vi "Trigger Pulse Width.vi"(5 "Lower Limit":dbl, 6 "Upper Limit":dbl, 7 "Type":i32(ring) caption="Mode" items=["Inside Limits", "Outside Limits", "Less Than", "Greater Than", "Equal To", "Not Equal To"], 8 "error in":errorcluster, 9 "Level":dbl, 10 "Source":i32(ring) items=["TTL0", "TTL1", "TTL2", "TTL3", "TTL4", "TTL5", "TTL6", "TTL7", "ECL0", "ECL1", "Input Channel 1", "Input Channel 2", "Input Channel 3", "Input Channel 4", "Eternal Trigger Source", "STAR", "Manual Trigger", "Pattern"], 11 "Instrument Handle In":i32) -> (0 "error out":errorcluster, 3 "Instrument Handle Out":i32)   [LabVIEW 8.6, in "ZTScopeM.lvlib"]
doc: "Set the trigger type to pulse width and configure the pulse width trigger settings."
uses:
  ZTScopeM.lvlib
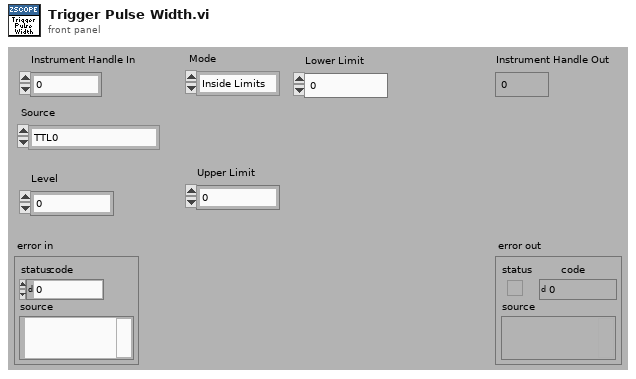
[diagram p1: front panel]
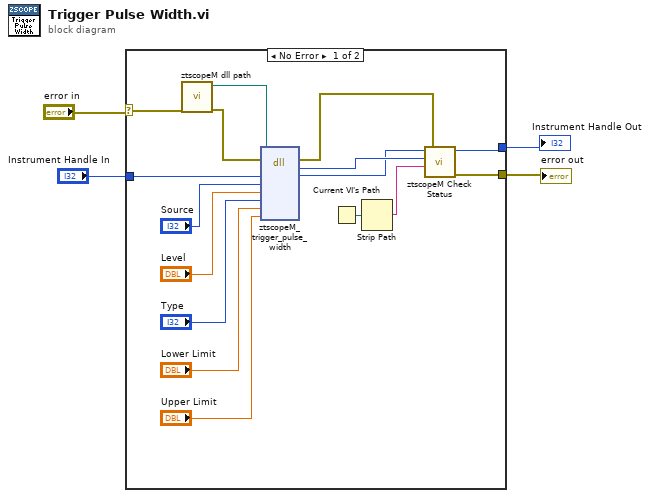
[diagram p0: block diagram]
diagram:
  n1 = case shown="No Error" "error in" {
    selector: "error in" -> [w8 w22]
    tunnel: [w9 w22] -> w2
    tunnel: "Instrument Handle In" -> [w20 w21]
    tunnel: [w10 w21] -> w1
    frame #0 {
      n2 = call "ztscopeM dll path.vi"("error in (no error)"=w8) -> ("error out"=w6:errorcluster, "<instrument>.dll path"=w7:path)  [unwired: 9 in]
      n3 = dll-call lib="C:/Program Files (x86)/National Instruments/LabVIEW 2013/instr.lib/ztscopem/ztscopeM.dll" fn="ztscopeM_trigger_pulse_width"(path in=w7, error in=w6, "instrumentHandle"=w20, "source"="Source", "level"="Level", "type"="Type", "lowerLimit"="Lower Limit", "upperLimit"="Upper Limit") -> (error out=w5:errorcluster, w12:i32, "instrumentHandle"=w11:i32)  [unwired: 6 in, 1 out]
      n4 = Current VI's Path() -> (path=w14:path)
      n5 = Strip Path(path=w14) -> (name=w13:string)  [unwired: 1 out]
      n6 = call "ztscopeM Check Status.vi"("error in"=w5, "name of VI"=w13, "status (return code)"=w12, "instrument handle in"=w11) -> ("error out"=w9:errorcluster, "instrument handle out"=w10:i32)  [unwired: 2 in]
    }
    frame #1 {
    }
  }
  "Instrument Handle Out" <- w1
  "error out" <- w2
